vi "运维调试界面.vi"() -> ()   [LabVIEW 2016, in "质控单元V4.lvlib"]
panel:
  in  "质控数据":T1
  in  "Tab Control 7":enum32{"参数"}(tab)
  out "CODmn运行流程":string caption="运行流程"
  in  "CODMn启用":bool caption="启用"
  out "CODMn剩余时间":string caption="剩余时间"
  out "CODMn当前步骤":string caption="当前步骤"
  out "CODMn当前流程":string caption="当前流程"
  out "CODMn告警状态":string caption="告警状态"
  out "CODMn液位状态":string caption="液位状态"
  out "CODMn运行状态":string caption="运行状态"
  out "CODMn通讯状态":bool caption="状态"
  in  "Tab Control 6":enum32{"参数"}(tab)
  out "总氮运行流程":string caption="运行流程"
  in  "总氮启用":bool caption="启用"
  out "TN剩余时间":string caption="剩余时间"
  out "TN当前步骤":string caption="当前步骤"
  out "TN当前流程":string caption="当前流程"
  out "TN告警状态":string caption="告警状态"
  out "TN液位状态":string caption="液位状态"
  out "TN运行状态":string caption="运行状态"
  out "TN通讯状态":bool caption="状态"
  in  "Tab Control 5":enum32{"参数"}(tab)
  out "总磷运行流程":string caption="运行流程"
  in  "总磷启用":bool caption="启用"
  out "TP剩余时间":string caption="剩余时间"
  out "TP当前步骤":string caption="当前步骤"
  out "TP当前流程":string caption="当前流程"
  out "TP告警状态":string caption="告警状态"
  out "TP液位状态":string caption="液位状态"
  out "TP运行状态":string caption="运行状态"
  out "TP通讯状态":bool caption="状态"
  in  "Tab Control 4":enum32{"参数"}(tab)
  out "氨氮剩余时间":string caption="剩余时间"
  out "氨氮当前步骤":string caption="当前步骤"
  out "氨氮当前流程":string caption="当前流程"
  out "氨氮告警状态":string caption="告警状态"
  out "氨氮液位状态":string caption="液位状态"
  out "氨氮运行状态":string caption="运行状态"
  out "氨氮通讯状态":bool caption="状态"
  in  "氨氮启用":bool caption="启用"
  out "氨氮运行流程":string caption="运行流程"
  in  "停止":bool
  in  "Slave ID":T2
  in  "参数设置":bool
  in  "串口设置":bool
  in  "调试界面":bool
  in  "加标回收":bool
  # "CODMn质控状态"
  # "总氮质控状态"
  # "总磷质控状态"
  # "氨氮质控状态"
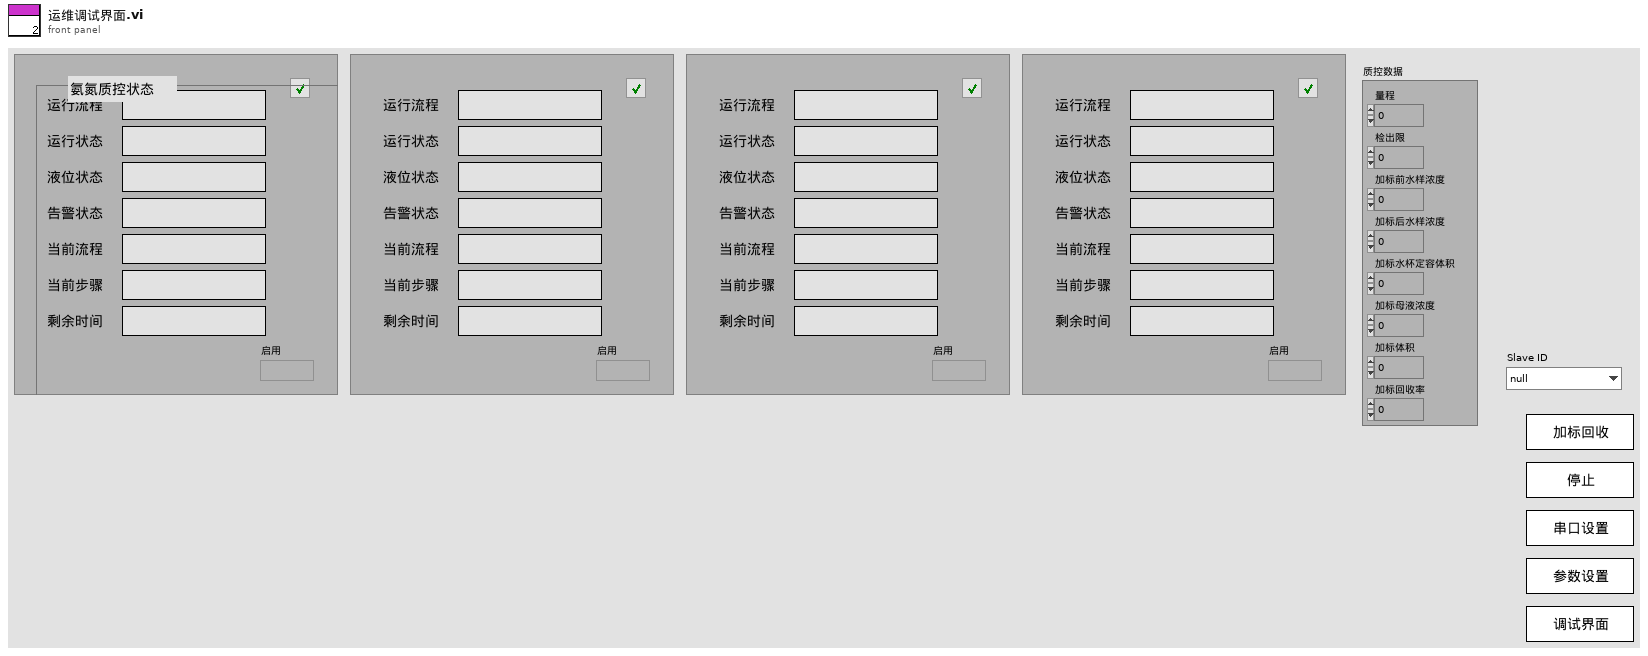
[diagram p1: front panel]
types:
  T1 = cluster{"量程":dbl, "检出限":dbl, "加标前水样浓度":dbl, "加标后水样浓度":dbl, "加标水杯定容体积":dbl, "加标母液浓度":dbl, "加标体积":dbl, "加标回收率":dbl}
  T2 = typedef "质控单元V4.lvlib/质控slave id.ctl" = enum16{"null", "氨氮", "总磷", "总氮", "CODMn", "CODCr", "氨氮总磷", "总磷总氮"}
  T3 = cluster{"氨氮":bool, "总磷":bool, "总氮":bool, "CODMn":bool, "CODCr":bool, "氨氮总磷":bool, "总磷总氮":bool}
  T4 = typedef "质控单元V4.lvlib/质控仪器状态显示.ctl" = cluster{"运行状态":string, "液位状态":string, "告警状态":string, "当前流程":string, "当前步骤":string, "剩余时间":string}
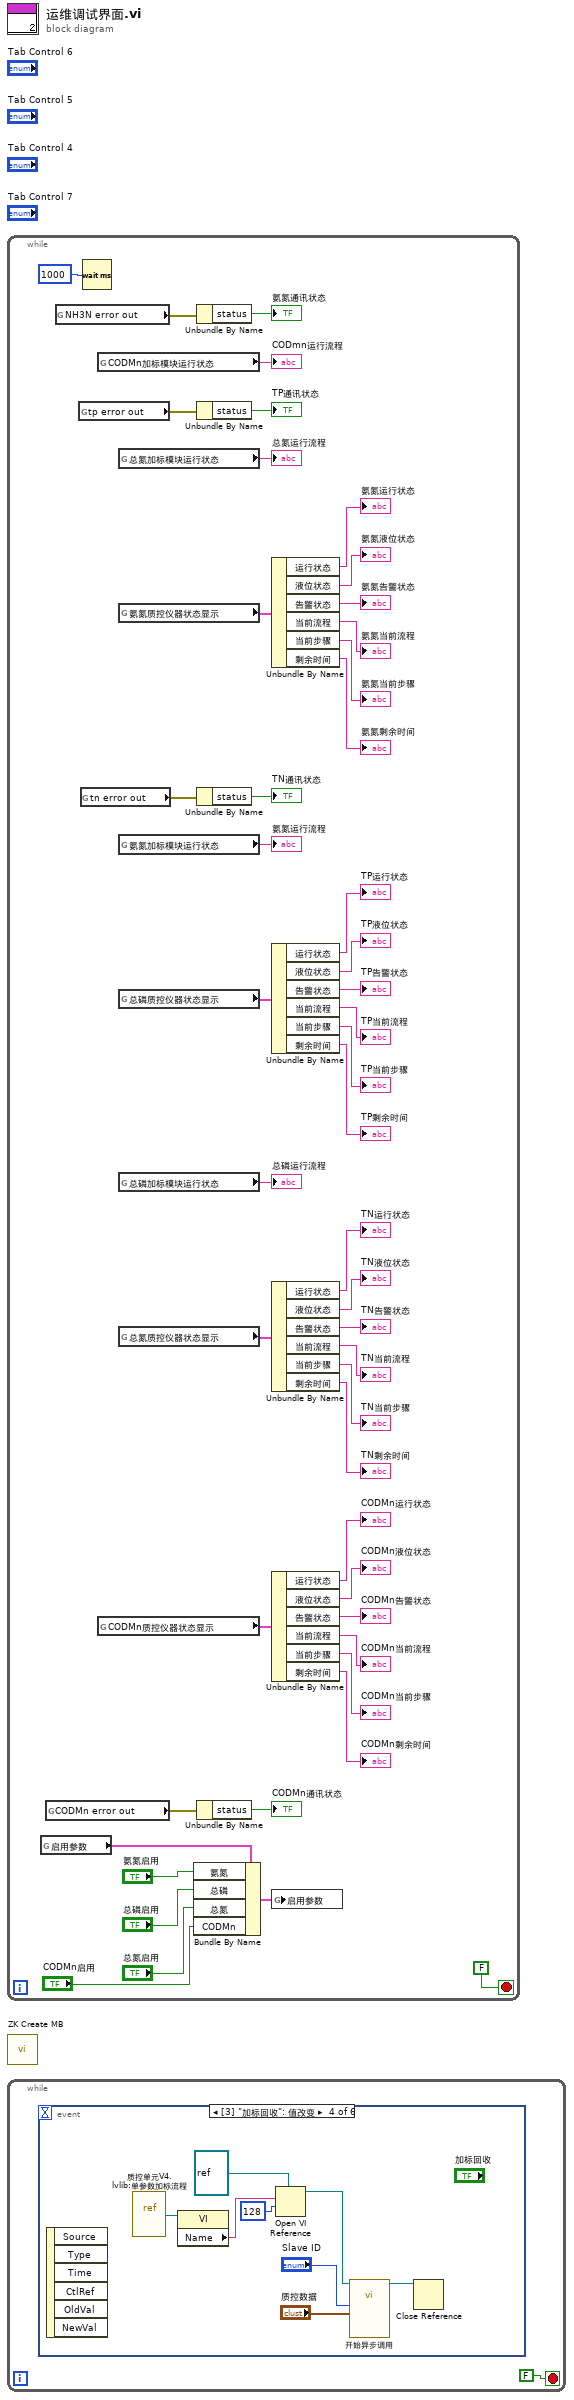
[diagram p0: block diagram]
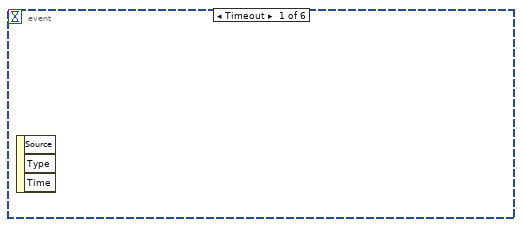
[diagram p2: hidden frame]
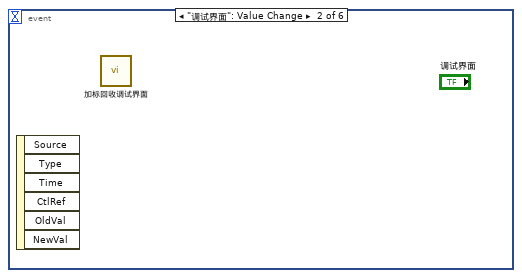
[diagram p3: hidden frame]
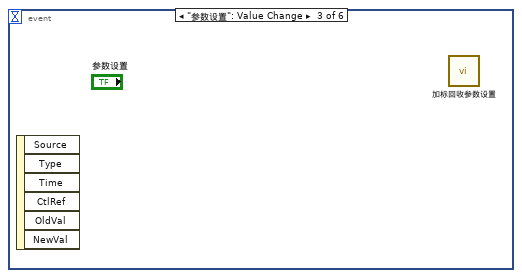
[diagram p4: hidden frame]
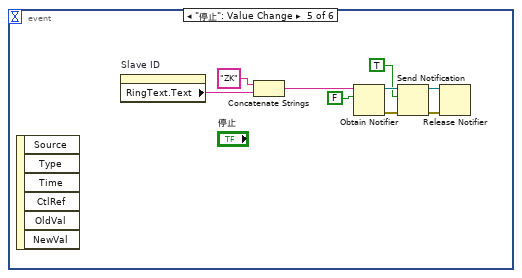
[diagram p5: hidden frame]
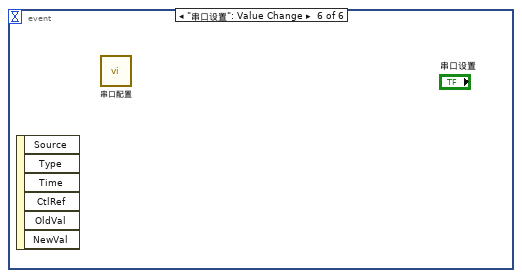
[diagram p6: hidden frame]
diagram:
  n1 = while {
    stop <- FALSE stop-if-true
    n2 = global read "ZK断电保存全局变量.vi" "启用参数"() -> (w7:T3)
    n3 = global read "ZK非断电保存全局变量.vi" "CODMn error out"() -> (w46:errorcluster)
    n4 = global read "ZK非断电保存全局变量.vi" "NH3N error out"() -> (w45:errorcluster)
    n5 = global read "ZK非断电保存全局变量.vi" "tp error out"() -> (w14:errorcluster)
    n6 = global read "ZK非断电保存全局变量.vi" "tn error out"() -> (w13:errorcluster)
    n7 = Wait (ms)(milliseconds to wait=u32 1000 ("等待时间（毫秒）")) -> ()  [unwired: 1 out]
    n8 = global read "ZK非断电保存全局变量.vi" "CODMn加标模块运行状态"() -> (→"CODmn运行流程":string)
    n9 = global read "ZK非断电保存全局变量.vi" "CODMn质控仪器状态显示"() -> (w22:T4)
    n10 = global read "ZK非断电保存全局变量.vi" "总氮加标模块运行状态"() -> (→"总氮运行流程":string)
    n11 = global read "ZK非断电保存全局变量.vi" "氨氮质控仪器状态显示"() -> (w43:T4)
    n12 = global read "ZK非断电保存全局变量.vi" "氨氮加标模块运行状态"() -> (→"氨氮运行流程":string)
    n13 = global read "ZK非断电保存全局变量.vi" "总磷质控仪器状态显示"() -> (w36:T4)
    n14 = global read "ZK非断电保存全局变量.vi" "总磷加标模块运行状态"() -> (→"总磷运行流程":string)
    n15 = global read "ZK非断电保存全局变量.vi" "总氮质控仪器状态显示"() -> (w29:T4)
    n16 = Bundle By Name(cluster=w7, "氨氮"="氨氮启用", "总磷"="总磷启用", "总氮"="总氮启用", "CODMn"="CODMn启用") -> (w6:T3)
    n17 = Unbundle By Name(w45) -> ("status"=→"氨氮通讯状态":bool)
    n18 = Unbundle By Name(w14) -> ("status"=→"TP通讯状态":bool)
    n19 = Unbundle By Name(w13) -> ("status"=→"TN通讯状态":bool)
    n20 = Unbundle By Name(w46) -> ("status"=→"CODMn通讯状态":bool)
    n21 = Unbundle By Name(w43) -> ("运行状态"=→"氨氮运行状态":string, "液位状态"=→"氨氮液位状态":string, "告警状态"=→"氨氮告警状态":string, "当前流程"=→"氨氮当前流程":string, "当前步骤"=→"氨氮当前步骤":string, "剩余时间"=→"氨氮剩余时间":string)
    n22 = Unbundle By Name(w36) -> ("运行状态"=→"TP运行状态":string, "液位状态"=→"TP液位状态":string, "告警状态"=→"TP告警状态":string, "当前流程"=→"TP当前流程":string, "当前步骤"=→"TP当前步骤":string, "剩余时间"=→"TP剩余时间":string)
    n23 = Unbundle By Name(w29) -> ("运行状态"=→"TN运行状态":string, "液位状态"=→"TN液位状态":string, "告警状态"=→"TN告警状态":string, "当前流程"=→"TN当前流程":string, "当前步骤"=→"TN当前步骤":string, "剩余时间"=→"TN剩余时间":string)
    n24 = Unbundle By Name(w22) -> ("运行状态"=→"CODMn运行状态":string, "液位状态"=→"CODMn液位状态":string, "告警状态"=→"CODMn告警状态":string, "当前流程"=→"CODMn当前流程":string, "当前步骤"=→"CODMn当前步骤":string, "剩余时间"=→"CODMn剩余时间":string)
    n25 = global write "ZK断电保存全局变量.vi" "启用参数"(w6) -> ()
  }
  n26 = call "ZK Create MB.vi"() -> ()  [unwired: 12 in]
  n27 = while {
    stop <- FALSE stop-if-true
    n28 = event shown="[3] \"加标回收\": 值改变" {
      selector: _ -> [_ _ _ _ _ _]
      dyn-events: _ -> [_ _ _ _ _ _]
      timeout: _ -> [_ _ _ _ _ _]
      event Timeout {
        n29 = event-data() -> ()  [unwired: 1 in, 3 out]
      }
      event "调试界面": Value Change {
        n30 = event-data() -> ()  [unwired: 1 in, 6 out]
        n31 = call "加标回收调试界面.vi"() -> ()  [unwired: 12 in]
      }
      event "参数设置": Value Change {
        n32 = event-data() -> ()  [unwired: 1 in, 6 out]
        n33 = call "加标回收参数设置.vi"() -> ()  [unwired: 12 in]
      }
      event "加标回收": Value Change {
        n34 = event-data() -> ()  [unwired: 1 in, 6 out]
        n35 = vi-ref "质控单元V4.lvlib:单参数加标流程.vi"() -> (w57:refnum<vi>)
        n36 = property class="VI"(reference=w57) -> ("Name"=w56:string)  [unwired: 1 in, 2 out]
        n37 = Open VI Reference(type specifier VI Refnum (for type only)=refnum<vi> refnum, vi path=w56, options=128 ("选项")) -> (vi reference=w53:refnum<vi>)  [unwired: 3 in, 1 out]
        n38 = call-by-ref "开始异步调用"(reference=w53, "质控数据"="质控数据", "Slave ID"="Slave ID") -> (reference out=w51:refnum<vi>)  [unwired: 11 in, 1 out]
        n39 = Close Reference(reference=w51) -> ()  [unwired: 1 in, 1 out]
      }
      event "停止": Value Change {
        n40 = event-data() -> ()  [unwired: 1 in, 6 out]
        n41 = property on="Slave ID" class="Enum (严格)"() -> ("RingText.Text"=w64:string)  [unwired: 2 in, 2 out]
        n42 = Concatenate Strings("ZK" ("名称（未命名）"), w64) -> (w63:string)
        n43 = Obtain Notifier(name (unnamed)=w63, notification data type=FALSE) -> (notifier out=w62:refnum<notifier>, error out=w61:errorcluster)  [unwired: 2 in, 1 out]
        n44 = Send Notification(notification=TRUE ("通知"), notifier=w62, error in (no error)=w61) -> (notifier out=w60:refnum<notifier>, error out=w59:errorcluster)
        n45 = Release Notifier(notifier=w60, error in (no error)=w59) -> ()  [unwired: 1 in, 3 out]
      }
      event "串口设置": Value Change {
        n46 = event-data() -> ()  [unwired: 1 in, 6 out]
        n47 = call "串口配置.vi"() -> ()  [unwired: 12 in]
      }
    }
  }
